vi "cm_Level Color Peak Read.vi"(4 "error in (no error)":errorcluster, 6 "Container State":T3, 7 "Display State In":T1={"Chan"=[], "First Drop?"=FALSE, "Notifier Name"="", "Refresh View"=FALSE, "Scale to Input Range"=FALSE, "Linear View"=FALSE, "Display"={"Current"=6618880, "Peak"=6618880}, "Property/Method"=enum."No Update", "Time Display Ref"=[]}) -> (0 "error out":errorcluster, 2 "Value":u32(colorbox)=6618880, 3 "Display State Out":T1={"Chan"=[], "First Drop?"=FALSE, "Notifier Name"="", "Refresh View"=FALSE, "Scale to Input Range"=FALSE, "Linear View"=FALSE, "Display"={"Current"=6618880, "Peak"=6618880}, "Property/Method"=enum."No Update", "Time Display Ref"=[]})   [LabVIEW 2012, in "Channel Monitor.xctl"]
doc: "Get the color of the peak bar."
uses:
  Channel Monitor.xctl
  <vilib>/_xctls/Container State.ctl
  subVIs/cm_Channel Monitor State.ctl
  TypeDef/cm_Property_Method.ctl
  <vilib>/_xctls/XControlSupport.lvlib
panel:
  # "Replace the Value Indicator below with an Indicator of desired type.\nDo not remove this Indicator or the others from the connector pane. \nDo not change the connector pane pattern.\nThe Value Indicator should always be the second terminal from top on the output side in the connector pane."
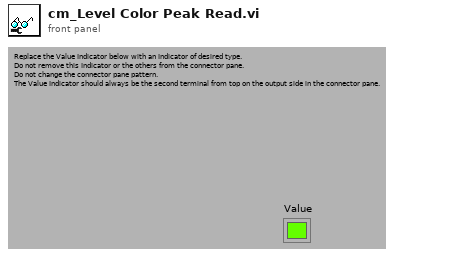
[diagram p1: front panel]
types:
  T1 = typedef "Channel Monitor.xctl/cm_Channel Monitor State.ctl" = cluster{"Chan":cluster{"ChanName":string, "Current":dbl, "Peak":dbl, "Input Range":dbl}[], "First Drop?":bool, "Notifier Name":string, "Refresh View":bool, "Scale to Input Range":bool, "Linear View":bool, "Display":cluster{"Current":u32, "Peak":u32}, "Property/Method":T2, "Time Display Ref":refnum<vi>[]}
  T2 = typedef "Channel Monitor.xctl/cm_Property_Method.ctl" = enum16{"No Update", "Color: Currrent", "Color: Peak", "Close Time Displays"}
  T3 = typedef "XControlSupport.lvlib/Container State.ctl" = cluster{"Indicator?":bool, "Run Mode?":bool, " Refnum":refnum<vi>}
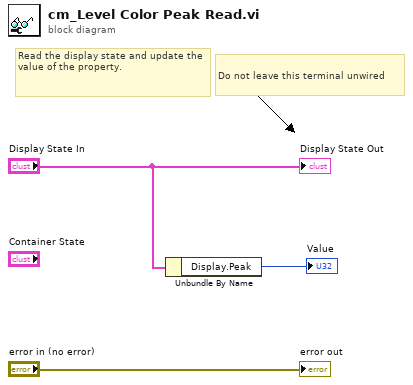
[diagram p0: block diagram]
diagram:
  # "Do not leave this terminal unwired"
  # "Read the display state and update the value of the property."
  n1 = Unbundle By Name("Display State In") -> ("Display.Peak"=→"Value":u32)
  "error out" <- "error in (no error)"
  "Display State Out" <- "Display State In"
